vi "3_sub_stringLine2array.vi"(11 "String":string) -> (3 "Array":string[](array[string]))   [LabVIEW 2023, in "2022.lvlib"]
uses:
  2022.lvlib
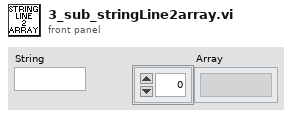
[diagram p1: front panel]
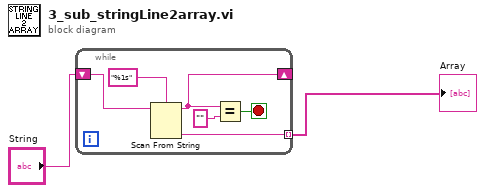
[diagram p0: block diagram]
diagram:
  n1 = while {
    shift-right: [w5] -> _
    shift-left: "String" -> [w8]
    tunnel: [w3] -> w1 mode=indexing
    stop <- w6 stop-if-true
    n2 = Scan From String(format string="%1s", input string=w8) -> (remaining string=w5:string, output 1=w3:string)  [unwired: 3 in, 2 out]
    n3 = Equal?(x=w5, y="") -> (x = y?=w6:bool)
  }
  "Array" <- w1
